vi "PRIME Telescope Parse Status Response.vi"(8 "error in":errorcluster, 10 "Reg List":string[](array[string])=["001", "002", "004", "007", "009", "011", "013", "015", "018", "019", "020", "021", "022", "025", "026", "027", "054", "078", "120", "306", "027"], 11 "input string":string) -> (0 "error out":errorcluster, 2 "msg timestamp":timestamp, 3 "Telescope Status":T1 {"Status Word" format="%x"})   [LabVIEW 2021, in "PRIME Telescope.lvclass"]
uses:
  PRIME Telescope.lvclass
  Telescope cluster Status.ctl
  typedefs/CC cluster RA and DEC.ctl
  Telescope enum Status.ctl
  <vilib>/regexp/Match Regular Expression.xnode
  Telescope.lvclass
panel:
  out "length":i32
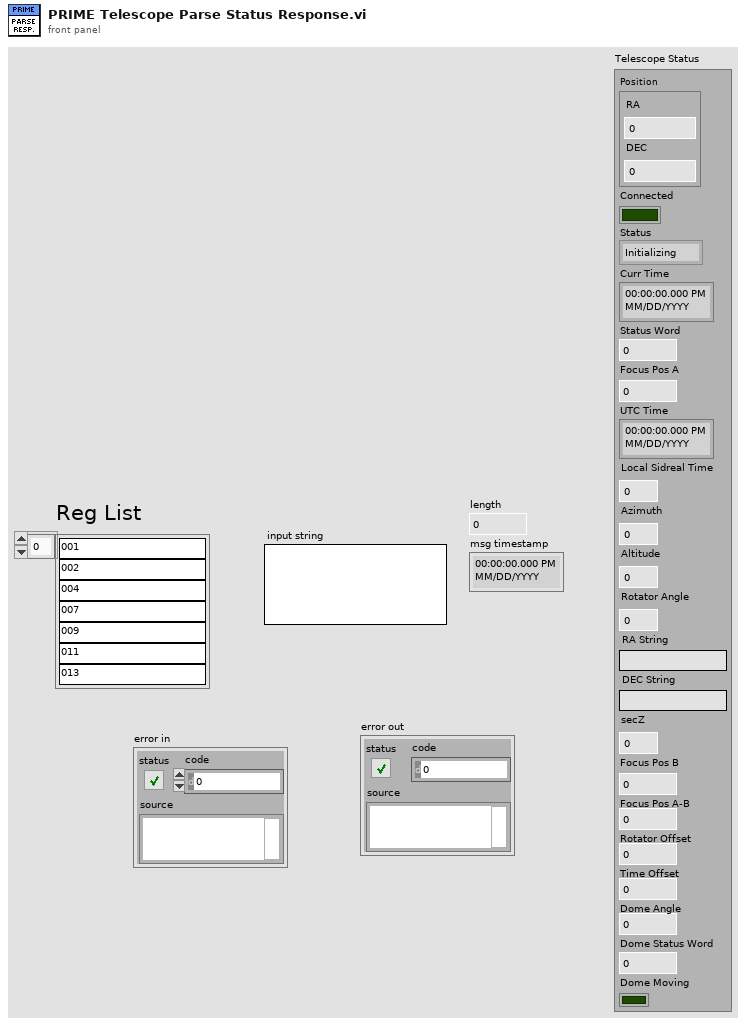
[diagram p1: front panel]
types:
  T1 = typedef "Telescope.lvclass/Telescope cluster Status.ctl" = cluster{"Position":T2, "Connected":bool, "Status":T3, "Curr Time":timestamp, "Status Word":u32, "Focus Pos A":dbl, "UTC Time":timestamp, "Local Sidreal Time":dbl, "Azimuth":dbl, "Altitude":dbl, "Rotator Angle":dbl, "RA String":string, "DEC String":string, "secZ":dbl, "Focus Pos B":dbl, "Focus Pos A-B":dbl, "Rotator Offset":dbl, "Time Offset":dbl, "Dome Angle":dbl, "Dome Status Word":u32, "Dome Moving":bool}
  T2 = typedef "CC cluster RA and DEC.ctl" = cluster{"RA":dbl, "DEC":dbl}
  T3 = typedef "Telescope.lvclass/Telescope enum Status.ctl" = enum16{"Initializing", "Ready", "Moving", "Focusing", "Error"}
  T4 = typedef "LVDateTimeRec.ctl" = cluster{"fractional second":dbl, "second":i32, "minute":i32, "hour":i32, "day of month":i32, "month":i32, "year":i32, "day of week":i32, "day of year":i32, "DST":i32}
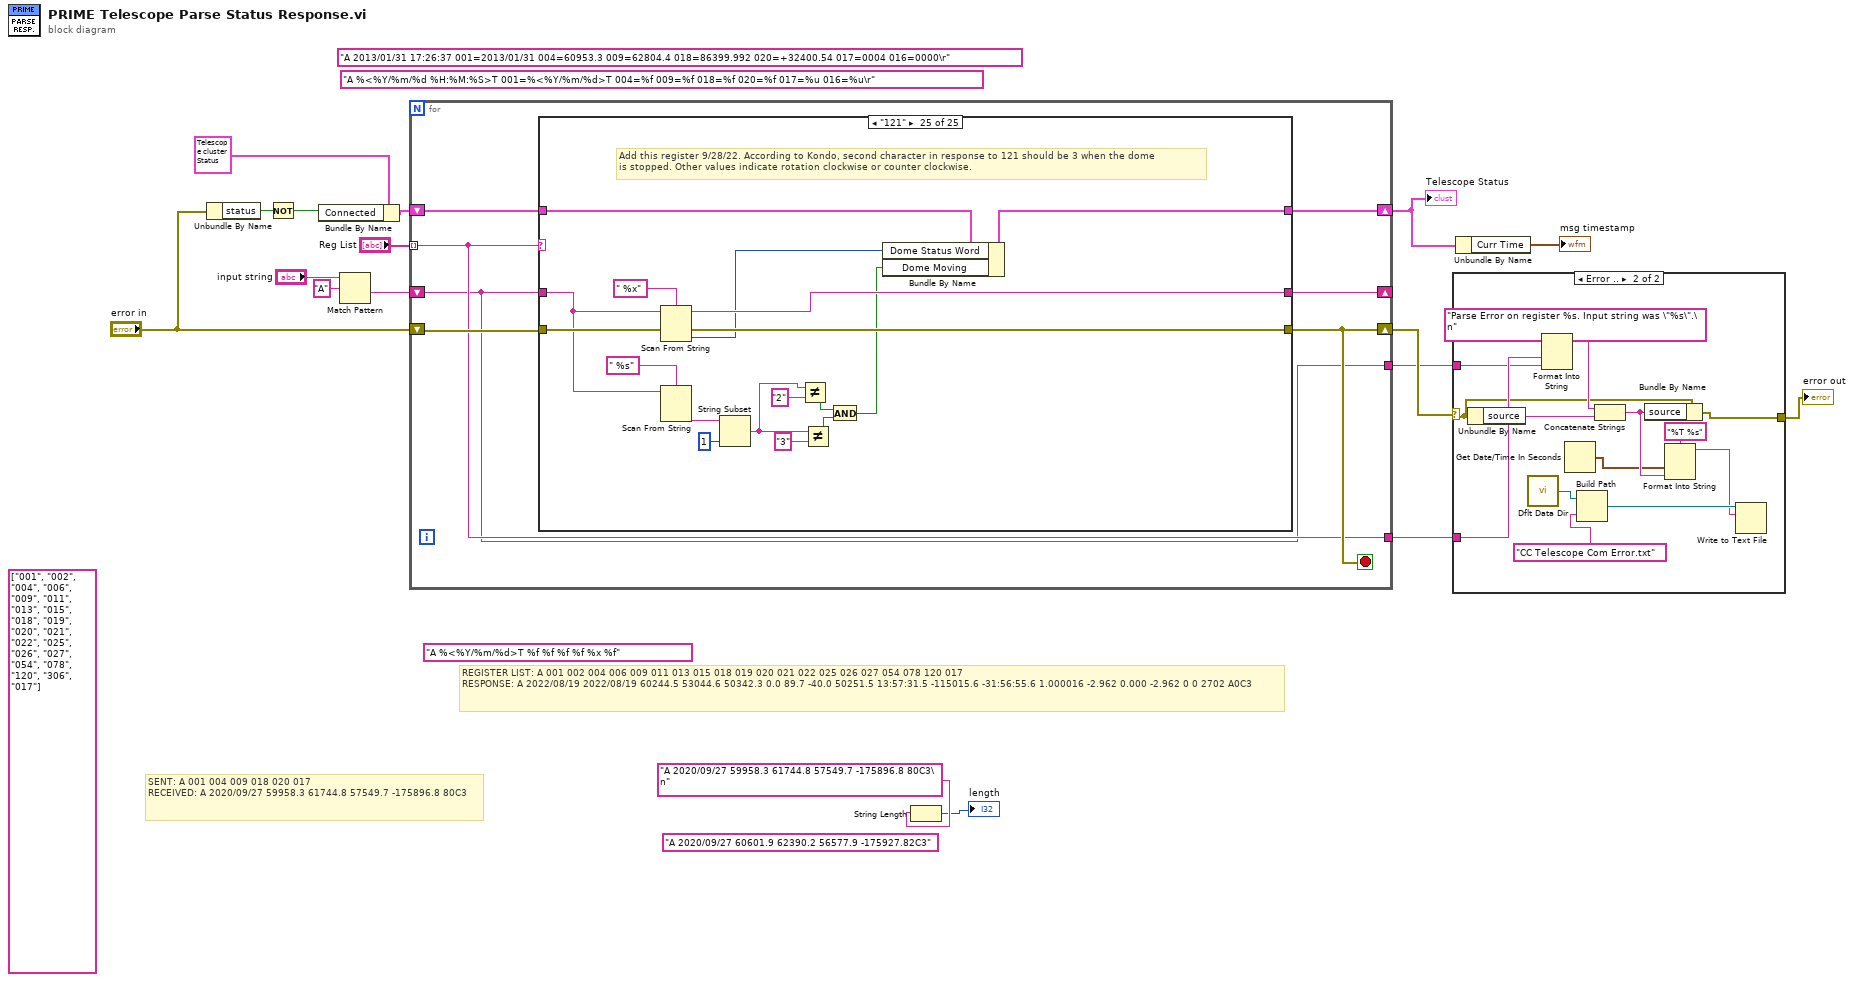
[diagram p0: block diagram]
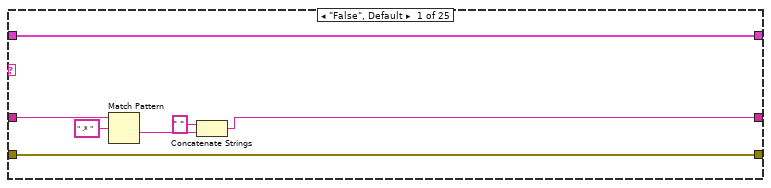
[diagram p3: hidden frame]
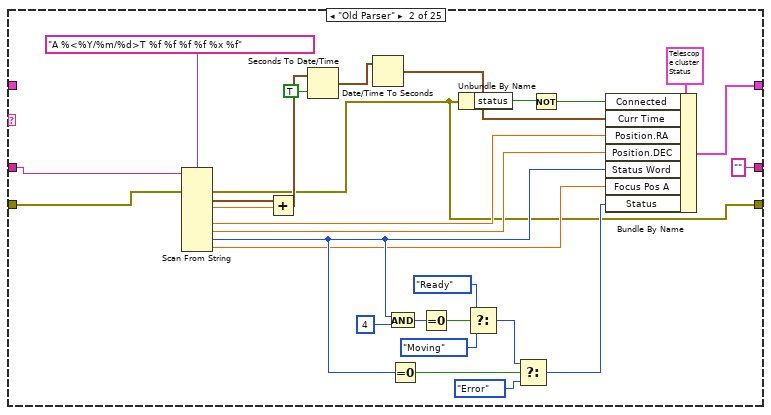
[diagram p4: hidden frame]
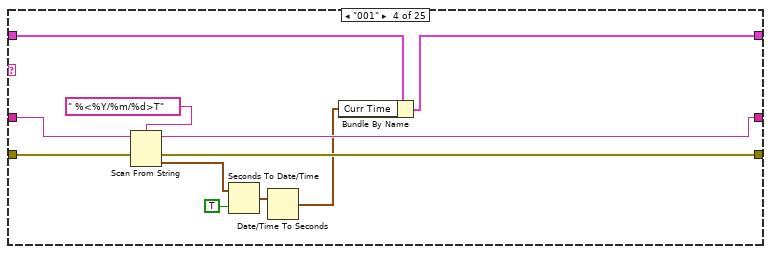
[diagram p6: hidden frame]
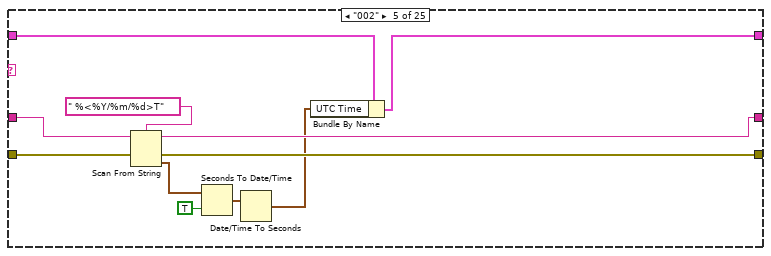
[diagram p7: hidden frame]
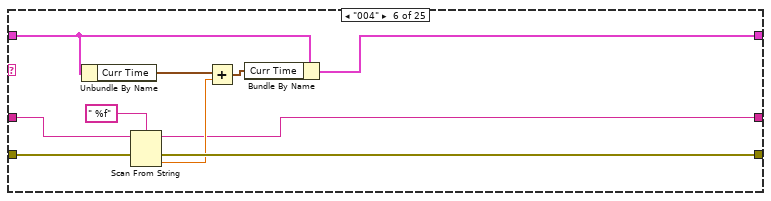
[diagram p8: hidden frame]
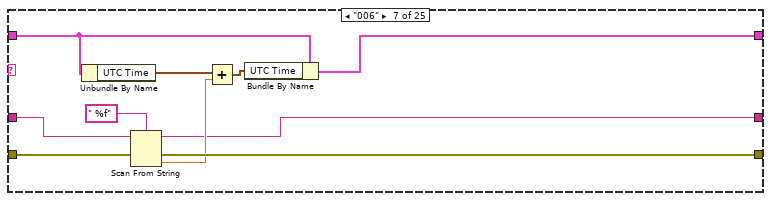
[diagram p9: hidden frame]
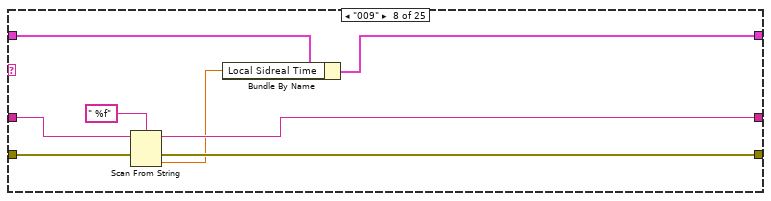
[diagram p10: hidden frame]
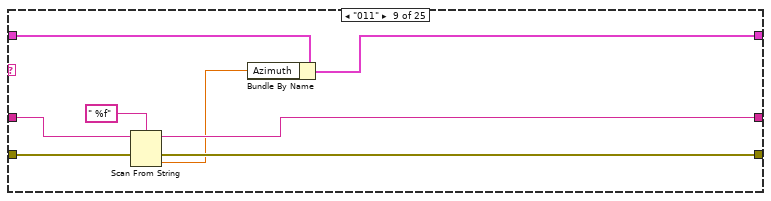
[diagram p11: hidden frame]
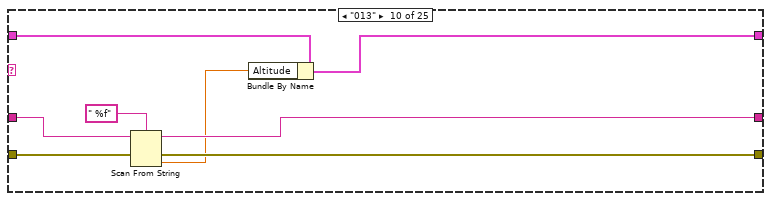
[diagram p12: hidden frame]
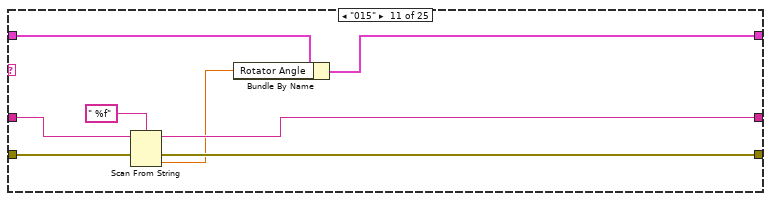
[diagram p13: hidden frame]
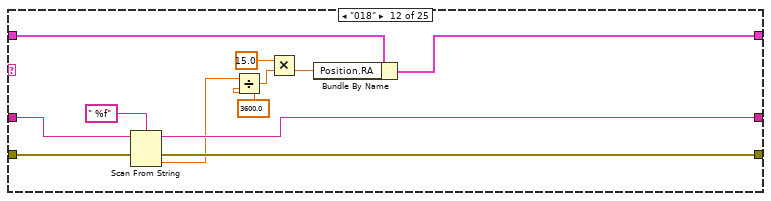
[diagram p14: hidden frame]
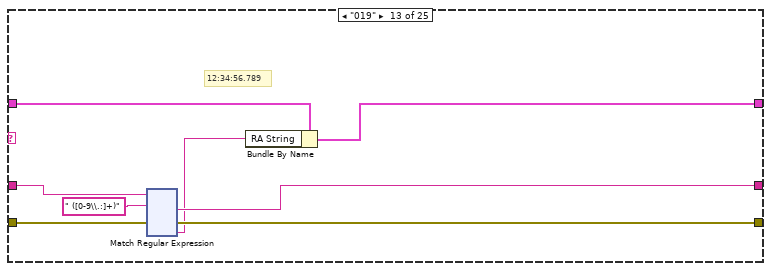
[diagram p15: hidden frame]
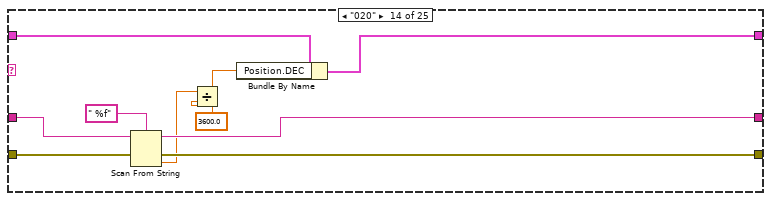
[diagram p16: hidden frame]
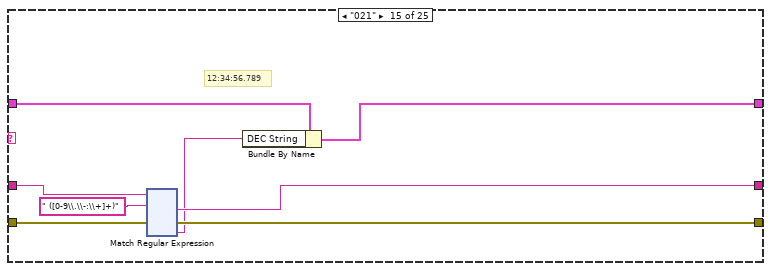
[diagram p17: hidden frame]
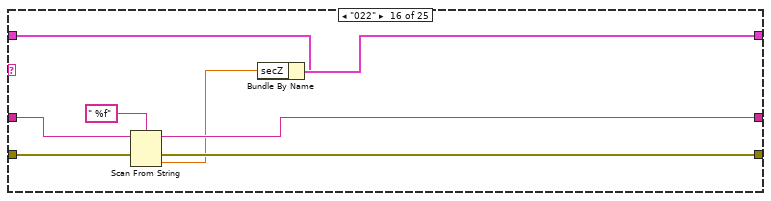
[diagram p18: hidden frame]
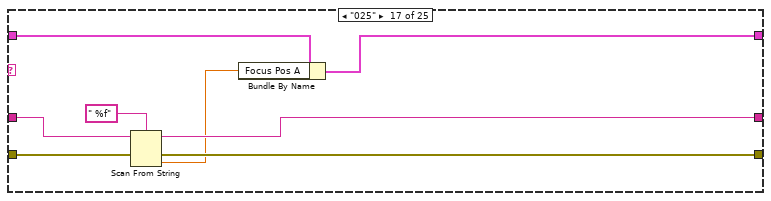
[diagram p19: hidden frame]
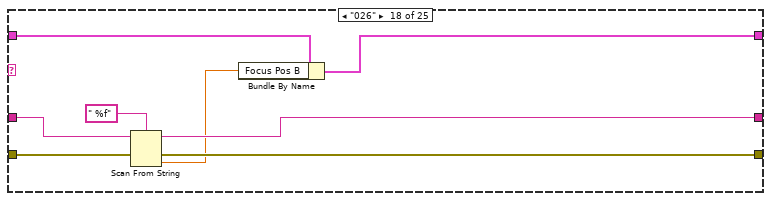
[diagram p20: hidden frame]
diagram:
  (unwired) "A %<%Y/%m/%d>T %f %f %f %f %x %f" ("format string")
  (unwired) string[] ["001", "002", "004", "006", "009", "011", "013", "015", "018", "019", "020", "021", "022", "025", "026", "027", "054", "078", "120", "306", "017"]
  (unwired) "A %<%Y/%m/%d %H:%M:%S>T 001=%<%Y/%m/%d>T 004=%f 009=%f 018=%f 020=%f 017=%u 016=%u\r" ("format string")
  (unwired) "A 2020/09/27 60601.9 62390.2 56577.9 -175927.82C3"
  (unwired) "A 2013/01/31 17:26:37 001=2013/01/31 004=60953.3 009=62804.4 018=86399.992 020=+32400.54 017=0004 016=0000\r" ("format string")
  # "REGISTER LIST: A 001 002 004 006 009 011 013 015 018 019 020 021 022 025 026 027 054 078 120 017\nRESPONSE: A 2022/08/19 2022/08/19 60244.5 53044.6 50342.3 0.0 89.7 -40.0 50251.5 13:57:31.5 -115015.6 -31:56:55.6 1.000016 -2.962 0.000 -2.962 0 0 2702 A0C3"
  # "SENT: A 001 004 009 018 020 017\nRECEIVED: A 2020/09/27 59958.3 61744.8 57549.7 -175896.8 80C3"
  n1 = Unbundle By Name("error in") -> ("status"=w8:bool)
  n2 = Not(x=w8) -> (.not. x?=w7:bool)
  n3 = Bundle By Name(cluster=T1 {"Position"={"RA"=0.0, "DEC"=0.0}, "Connected"=FALSE, "Status"=enum."Initializing", "Curr Time"=timestamp(0 s since 1904-01-01), "Status Word"=0, "Focus Pos A"=0.0, "UTC Time"=timestamp(0 s since 1904-01-01), "Local Sidreal Time"=0.0, "Azimuth"=0.0, "Altitude"=0.0, "Rotator Angle"=0.0, "RA String"="", "DEC String"="", "secZ"=0.0, "Focus Pos B"=0.0, "Focus Pos A-B"=0.0, "Rotator Offset"=0.0, "Time Offset"=0.0, "Dome Angle"=0.0, "Dome Status Word"=0, "Dome Moving"=FALSE} ("Telescope Status"), "Connected"=w7) -> (w10:T1)
  n4 = Match Pattern(string="input string", regular expression="A") -> (after substring=w12:string)  [unwired: 1 in, 3 out]
  n5 = for {
    tunnel: "Reg List" -> [w19] mode=indexing
    shift-right: [w24] -> w6
    shift-left: w10 -> [w23]
    shift-right: [w22] -> _
    shift-left: w12 -> [w18]
    shift-right: [w20] -> w4
    shift-left: "error in" -> [w21]
    tunnel: [w19] -> w2
    tunnel: [w18] -> w1
    stop <- w20 stop-if-true
    n6 = case shown="\"121\"" w19 {
      tunnel: [w31 w57 w62 w69 w80 w91 w101 w109 w117 w125 w133 w145 w156 w282 w293 w417 w425 w433 w441 w449 w457 w467 w471 w495 w512] -> w24
      tunnel: w21 -> [w25 w47 w60 w71 w82 w92 w102 w110 w118 w126 w134 w146 w153 w283 w290 w418 w426 w434 w442 w450 w458 w468 w475 w496 w513]
      tunnel: w18 -> [w30 w34 w61 w72 w83 w93 w103 w111 w119 w127 w135 w147 w151 w284 w288 w419 w427 w435 w443 w451 w459 w469 w476 w488 w507]
      tunnel: w23 -> [w31 _ w62 w70 w81 w89 w99 w107 w115 w123 w131 w143 w155 w280 w292 w415 w423 w431 w439 w447 w455 w465 w471 w486 w510]
      tunnel: [w25 w33 w60 w68 w79 w90 w100 w108 w116 w124 w132 w144 w152 w281 w289 w416 w424 w432 w440 w448 w456 w466 w474 w494 w511] -> w20
      tunnel: [w26 "" ("after match") w61 w67 w78 w85 w95 w106 w114 w122 w130 w142 w150 w279 w287 w414 w422 w430 w438 w446 w454 w464 w473 w493 w509] -> w22
      frame "False", Default {
        n7 = Match Pattern(string=w30, regular expression=" .* ") -> (after substring=w28:string)  [unwired: 1 in, 3 out]
        n8 = Concatenate Strings(" " ("string"), w28) -> (w26:string)
      }
      frame "Old Parser" {
        n9 = Scan From String(format string="A %<%Y/%m/%d>T %f %f %f %f %x %f", input string=w34, error in=w47) -> (error out=w33:errorcluster, output 1=w44:timestamp, output 2=w43:dbl, output 4=w42:dbl, output 5=w41:dbl, output 6=w40:u32, output 7=w35:dbl)  [unwired: 9 in, 2 out]
        n10 = Add(x=w44, y=w43) -> (x+y=w39:timestamp)
        n11 = Seconds To Date/Time(time stamp (now)=w39, to UTC (F)=TRUE) -> (date time rec=w37:T4)
        n12 = Date/Time To Seconds(2:w37) -> (0:w36:timestamp)  [unwired: 1 in]
        n13 = And(x=w40, y=u32 4) -> (x .and. y?=w55:u32)
        n14 = Equal To 0?(x=w40) -> (x = 0?=w51:bool)
        n15 = Equal To 0?(x=w55) -> (x = 0?=w54:bool)
        n16 = Unbundle By Name(w33) -> ("status"=w46:bool)
        n17 = Select(t=Telescope_enum_Status."Ready" ("Status"), s=w54, f=Telescope_enum_Status."Moving" ("Status")) -> (s? t:f=w50:T3)
        n18 = Select(t=w50, s=w51, f=Telescope_enum_Status."Error" ("Status")) -> (s? t:f=w48:T3)
        n19 = Not(x=w46) -> (.not. x?=w45:bool)
        n20 = Bundle By Name(cluster=T1 {"Position"={"RA"=0.0, "DEC"=0.0}, "Connected"=FALSE, "Status"=enum."Initializing", "Curr Time"=timestamp(0 s since 1904-01-01), "Status Word"=0, "Focus Pos A"=0.0, "UTC Time"=timestamp(0 s since 1904-01-01), "Local Sidreal Time"=0.0, "Azimuth"=0.0, "Altitude"=0.0, "Rotator Angle"=0.0, "RA String"="", "DEC String"="", "secZ"=0.0, "Focus Pos B"=0.0, "Focus Pos A-B"=0.0, "Rotator Offset"=0.0, "Time Offset"=0.0, "Dome Angle"=0.0, "Dome Status Word"=0, "Dome Moving"=FALSE} ("Telescope Status"), "Connected"=w45, "Curr Time"=w36, "Position.RA"=w42, "Position.DEC"=w41, "Status Word"=w40, "Focus Pos A"=w35, "Status"=w48) -> (w57:T1)
      }
      frame "error" {
      }
      frame "001" {
        n21 = Scan From String(format string=" %<%Y/%m/%d>T", input string=w72, error in=w71) -> (remaining string=w67:string, error out=w68:errorcluster, output 1=w65:timestamp)  [unwired: 2 in, 1 out]
        n22 = Seconds To Date/Time(time stamp (now)=w65, to UTC (F)=TRUE) -> (date time rec=w66:T4)
        n23 = Date/Time To Seconds(2:w66) -> (0:w63:timestamp)  [unwired: 1 in]
        n24 = Bundle By Name(cluster=w70, "Curr Time"=w63) -> (w69:T1)
      }
      frame "002" {
        n25 = Scan From String(format string=" %<%Y/%m/%d>T", input string=w83, error in=w82) -> (remaining string=w78:string, error out=w79:errorcluster, output 1=w75:timestamp)  [unwired: 2 in, 1 out]
        n26 = Seconds To Date/Time(time stamp (now)=w75, to UTC (F)=TRUE) -> (date time rec=w77:T4)
        n27 = Date/Time To Seconds(2:w77) -> (0:w74:timestamp)  [unwired: 1 in]
        n28 = Bundle By Name(cluster=w81, "UTC Time"=w74) -> (w80:T1)
      }
      frame "004" {
        n29 = Unbundle By Name(w89) -> ("Curr Time"=w88:timestamp)
        n30 = Scan From String(format string=" %f", input string=w93, error in=w92) -> (remaining string=w85:string, error out=w90:errorcluster, output 1=w87:dbl)  [unwired: 2 in, 1 out]
        n31 = Add(x=w88, y=w87) -> (x+y=w86:timestamp)
        n32 = Bundle By Name(cluster=w89, "Curr Time"=w86) -> (w91:T1)
      }
      frame "006" {
        n33 = Unbundle By Name(w99) -> ("UTC Time"=w98:timestamp)
        n34 = Scan From String(format string=" %f", input string=w103, error in=w102) -> (remaining string=w95:string, error out=w100:errorcluster, output 1=w97:dbl)  [unwired: 2 in, 1 out]
        n35 = Add(x=w98, y=w97) -> (x+y=w96:timestamp)
        n36 = Bundle By Name(cluster=w99, "UTC Time"=w96) -> (w101:T1)
      }
      frame "009" {
        n37 = Scan From String(format string=" %f", input string=w111, error in=w110) -> (remaining string=w106:string, error out=w108:errorcluster, output 1=w105:dbl)  [unwired: 2 in, 1 out]
        n38 = Bundle By Name(cluster=w107, "Local Sidreal Time"=w105) -> (w109:T1)
      }
      frame "011" {
        n39 = Scan From String(format string=" %f", input string=w119, error in=w118) -> (remaining string=w114:string, error out=w116:errorcluster, output 1=w113:dbl)  [unwired: 2 in, 1 out]
        n40 = Bundle By Name(cluster=w115, "Azimuth"=w113) -> (w117:T1)
      }
      frame "013" {
        n41 = Scan From String(format string=" %f", input string=w127, error in=w126) -> (remaining string=w122:string, error out=w124:errorcluster, output 1=w121:dbl)  [unwired: 2 in, 1 out]
        n42 = Bundle By Name(cluster=w123, "Altitude"=w121) -> (w125:T1)
      }
      frame "015" {
        n43 = Scan From String(format string=" %f", input string=w135, error in=w134) -> (remaining string=w130:string, error out=w132:errorcluster, output 1=w129:dbl)  [unwired: 2 in, 1 out]
        n44 = Bundle By Name(cluster=w131, "Rotator Angle"=w129) -> (w133:T1)
      }
      frame "018" {
        n45 = Scan From String(format string=" %f", input string=w147, error in=w146) -> (remaining string=w142:string, error out=w144:errorcluster, output 1=w140:dbl)  [unwired: 2 in, 1 out]
        n46 = Divide(x=w140, y=3600.0 ("x")) -> (x/y=w139:dbl)
        n47 = Multiply(x=15.0, y=w139) -> (x*y=w138:dbl)
        n48 = Bundle By Name(cluster=w143, "Position.RA"=w138) -> (w145:T1)
      }
      frame "019" {
        # "12:34:56.789"
        n49 = xnode "Match Regular Expression"("input string"=w151, "regular expression"=" ([0-9\\.:]+)", "error in"=w153) -> ("after match"=w150:string, "error out"=w152:errorcluster, "submatch 1"=w149:string)  [unwired: 3 in, 3 out]
        n50 = Bundle By Name(cluster=w155, "RA String"=w149) -> (w156:T1)
      }
      frame "020" {
        n51 = Scan From String(format string=" %f", input string=w284, error in=w283) -> (remaining string=w279:string, error out=w281:errorcluster, output 1=w278:dbl)  [unwired: 2 in, 1 out]
        n52 = Divide(x=w278, y=3600.0 ("x")) -> (x/y=w277:dbl)
        n53 = Bundle By Name(cluster=w280, "Position.DEC"=w277) -> (w282:T1)
      }
      frame "021" {
        # "12:34:56.789"
        n54 = xnode "Match Regular Expression"("input string"=w288, "regular expression"=" ([0-9\\.\\-:\\+]+)", "error in"=w290) -> ("after match"=w287:string, "error out"=w289:errorcluster, "submatch 1"=w286:string)  [unwired: 3 in, 3 out]
        n55 = Bundle By Name(cluster=w292, "DEC String"=w286) -> (w293:T1)
      }
      frame "022" {
        n56 = Scan From String(format string=" %f", input string=w419, error in=w418) -> (remaining string=w414:string, error out=w416:errorcluster, output 1=w413:dbl)  [unwired: 2 in, 1 out]
        n57 = Bundle By Name(cluster=w415, "secZ"=w413) -> (w417:T1)
      }
      frame "025" {
        n58 = Scan From String(format string=" %f", input string=w427, error in=w426) -> (remaining string=w422:string, error out=w424:errorcluster, output 1=w421:dbl)  [unwired: 2 in, 1 out]
        n59 = Bundle By Name(cluster=w423, "Focus Pos A"=w421) -> (w425:T1)
      }
      frame "026" {
        n60 = Scan From String(format string=" %f", input string=w435, error in=w434) -> (remaining string=w430:string, error out=w432:errorcluster, output 1=w429:dbl)  [unwired: 2 in, 1 out]
        n61 = Bundle By Name(cluster=w431, "Focus Pos B"=w429) -> (w433:T1)
      }
      frame "027" {
        n62 = Scan From String(format string=" %f", input string=w443, error in=w442) -> (remaining string=w438:string, error out=w440:errorcluster, output 1=w437:dbl)  [unwired: 2 in, 1 out]
        n63 = Bundle By Name(cluster=w439, "Focus Pos A-B"=w437) -> (w441:T1)
      }
      frame "054" {
        n64 = Scan From String(format string=" %f", input string=w451, error in=w450) -> (remaining string=w446:string, error out=w448:errorcluster, output 1=w445:dbl)  [unwired: 2 in, 1 out]
        n65 = Bundle By Name(cluster=w447, "Rotator Offset"=w445) -> (w449:T1)
      }
      frame "078" {
        n66 = Scan From String(format string=" %f", input string=w459, error in=w458) -> (remaining string=w454:string, error out=w456:errorcluster, output 1=w453:dbl)  [unwired: 2 in, 1 out]
        n67 = Bundle By Name(cluster=w455, "Time Offset"=w453) -> (w457:T1)
      }
      frame "120" {
        n68 = Scan From String(format string=" %f", input string=w469, error in=w468) -> (remaining string=w464:string, error out=w466:errorcluster, output 1=w463:dbl)  [unwired: 2 in, 1 out]
        n69 = Divide(x=w463, y=10.0 ("x")) -> (x/y=w462:dbl)
        n70 = Bundle By Name(cluster=w465, "Dome Angle"=w462) -> (w467:T1)
      }
      frame "306" {
        n71 = Scan From String(format string=" %f", input string=w476, error in=w475) -> (remaining string=w473:string, error out=w474:errorcluster, output 1=w472:dbl)  [unwired: 2 in, 1 out]
        n72 = Bundle By Name(cluster=w471, "Dome Angle"=w472) -> ()  [unwired: 1 out]
      }
      frame "017" {
        w480 = 1 ("offset (0)")
        # "Look only at the second character. If 0, not moving. Note that the \"Moving\" flag in the status word is true if trcaking is\non. So we use different logic to determine if the telescope is moving.\nThe telescope is ready iff (!Dome Moving) AND (Second character of status word == '0') \nMatches Japanese Python code. 9/28/22"
        n73 = Scan From String(format string=" %x", input string=w488, error in=w496) -> (remaining string=w493:string, error out=w494:errorcluster, output 1=w490:u32)  [unwired: 2 in, 1 out]
        n74 = Scan From String(format string=" %s", input string=w488) -> (output 1=w481:string)  [unwired: 3 in, 3 out]
        n75 = String Subset(string=w481, offset (0)=w480, length (rest)=w480) -> (substring=w479:string)
        n76 = Unbundle By Name(w486) -> ("Dome Moving"=w483:bool)
        n77 = Equal?(x="0", y=w479) -> (x = y?=w485:bool)
        n78 = Not(x=w483) -> (.not. x?=w484:bool)
        n79 = And(x=w484, y=w485) -> (x .and. y?=w482:bool)
        n80 = Select(t=Telescope_enum_Status."Ready" ("Status"), s=w482, f=Telescope_enum_Status."Moving" ("Status")) -> (s? t:f=w489:T3)
        n81 = Bundle By Name(cluster=w486, "Status Word"=w490, "Status"=w489) -> (w495:T1)
      }
      frame "121" {
        # "Add this register 9/28/22. According to Kondo, second character in response to 121 should be 3 when the dome\nis stopped. Other values indicate rotation clockwise or counter clockwise."
        n82 = Scan From String(format string=" %x", input string=w507, error in=w513) -> (remaining string=w509:string, error out=w511:errorcluster, output 1=w508:u32)  [unwired: 2 in, 1 out]
        n83 = Scan From String(format string=" %s", input string=w507) -> (output 1=w505:string)  [unwired: 3 in, 3 out]
        n84 = String Subset(string=w505, length (rest)=1 ("length (rest)")) -> (substring=w501:string)  [unwired: 1 in]
        n85 = Not Equal?(x=w501, y="2") -> (x != y?=w500:bool)
        n86 = Not Equal?(x=w501, y="3") -> (x != y?=w499:bool)
        n87 = And(x=w500, y=w499) -> (x .and. y?=w498:bool)
        n88 = Bundle By Name(cluster=w510, "Dome Status Word"=w508, "Dome Moving"=w498) -> (w512:T1)
      }
    }
  }
  "Telescope Status" <- w6
  n89 = String Length(string="A 2020/09/27 59958.3 61744.8 57549.7 -175896.8 80C3\n") -> (length=→"length":i32)
  n90 = case shown="Error .." w4 {
    selector: w4 -> [w515 w524]
    tunnel: [w515 w523] -> w3
    tunnel: w2 -> [_ w528]
    tunnel: w1 -> [_ w527]
    frame No Error {
    }
    frame Error {
      n91 = Unbundle By Name(w524) -> ("source"=w525:string)
      n92 = call <vilib>:"Dflt Data Dir.vi"() -> ("App:Default Data Directory"=w522:path)
      n93 = Format Into String(format string="Parse Error on register %s. Input string was \"%s\".\n", w528, w527) -> (resulting string=w526:string)  [unwired: 2 in, 1 out]
      n94 = Get Date/Time In Seconds() -> (seconds since 1Jan1904=w517:timestamp)
      n95 = Build Path(base path=w522, name or relative path="CC Telescope Com Error.txt") -> (appended path=w520:path)
      n96 = Concatenate Strings(w526, w525) -> (w518:string)
      n97 = Bundle By Name(cluster=w524, "source"=w518) -> (w523:errorcluster)
      n98 = Format Into String(format string="%T %s", w517, w518) -> (resulting string=w516:string)  [unwired: 2 in, 1 out]
      n99 = Write to Text File(file (use dialog)=w520, text=w516) -> ()  [unwired: 2 in, 3 out]
    }
  }
  "error out" <- w3
  n100 = Unbundle By Name(w6) -> ("Curr Time"=→"msg timestamp":timestamp)
